vi "Untitled 6 (SubVI).vi"(0 "Path":path, 1 "Dust ID":sgl, 5 "Upper Timestamp":timestamp, 7 "Velocity Limits":cluster{dbl, dbl}, 8 "Lower Timestamp":timestamp, 9 "Minimun Session Quality":i8, 13 "Use Timestamp":bool, 16 "Use Dust ID":bool, 17 "Dust Material":string) -> (20 "Results Output":string, 21 "Results Error/Debug":string, 25 "Request":string)   [LabVIEW 2015]
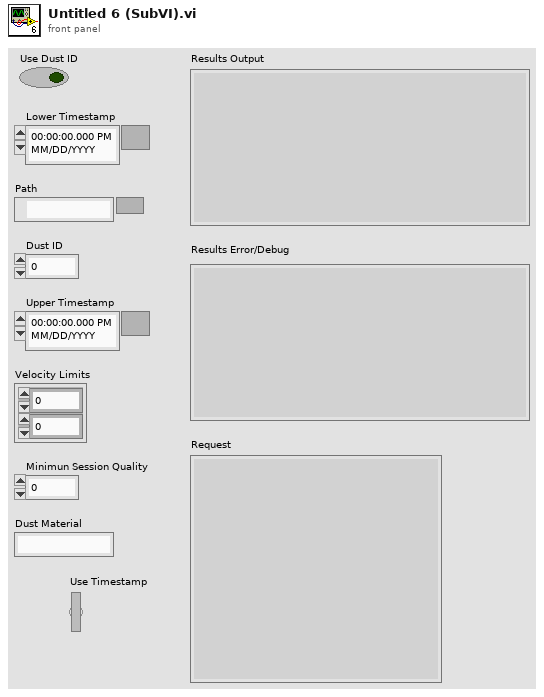
[diagram p1: front panel]
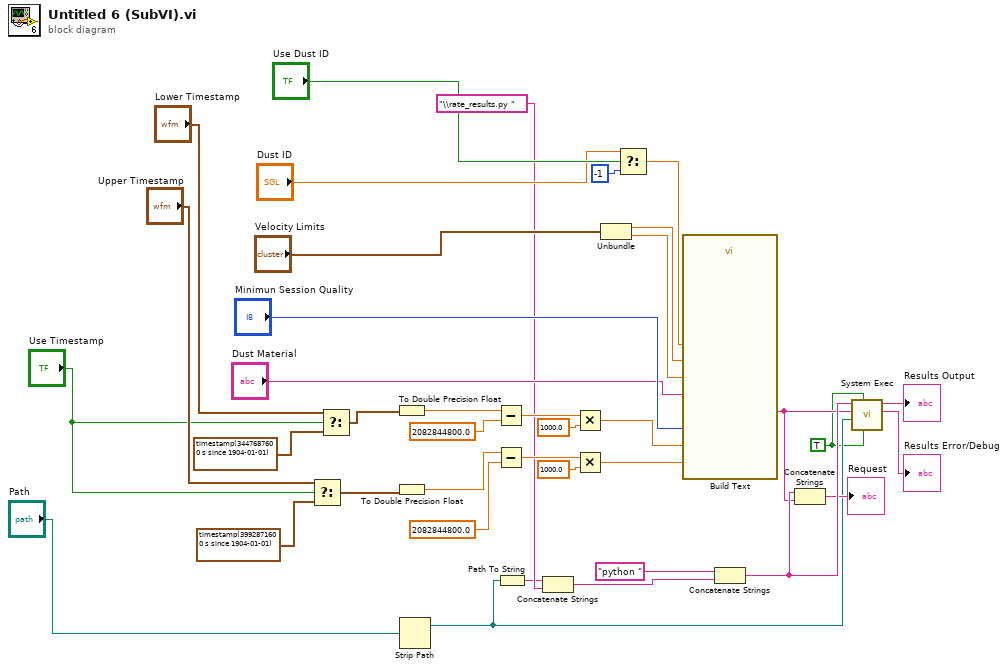
[diagram p0: block diagram]
diagram:
  w12 = TRUE
  n1 = Select(t="Upper Timestamp", s="Use Timestamp", f=timestamp(3992871600 s since 1904-01-01)) -> (s? t:f=w7:timestamp)
  n2 = Select(t="Lower Timestamp", s="Use Timestamp", f=timestamp(3447687600 s since 1904-01-01)) -> (s? t:f=w6:timestamp)
  n3 = To Double Precision Float(number=w6) -> (double precision float=w19:dbl)
  n4 = To Double Precision Float(number=w7) -> (double precision float=w15:dbl)
  n5 = Strip Path(path="Path") -> (stripped path=w13:path)  [unwired: 1 out]
  n6 = Subtract(x=w19, y=2082844800.0) -> (x-y=w21:dbl)
  n7 = Subtract(x=w15, y=2082844800.0) -> (x-y=w17:dbl)
  n8 = Path To String(path=w13) -> (string=w8:string)
  n9 = Concatenate Strings(w8, "\\rate_results.py ") -> (w11:string)
  n10 = Multiply(x=w21, y=1000.0) -> (x*y=w23:dbl)
  n11 = Multiply(x=w17, y=1000.0) -> (x*y=w24:dbl)
  n12 = Unbundle("Velocity Limits") -> (w26:dbl, w27:dbl)
  n13 = Select(t="Dust ID", s="Use Dust ID", f=-1) -> (s? t:f=w33:sgl)
  n14 = call "Build Text"("dustID"=w33, "vmax"=w27, "qual"="Minimun Session Quality", "start"=w23, "stop"=w24, "vmin"=w26, "material"="Dust Material") -> ("Result"=w35:string)  [unwired: 7 in, 1 out]
  n15 = Concatenate Strings("python ", w11) -> (w36:string)
  n16 = Concatenate Strings(w36, w35) -> (→"Request":string)
  n17 = call <vilib>:"System Exec.vi"("run minimized? (F)"=w12, "wait until completion? (T)"=w12, "working directory"=w13, "standard input"=w35, "command line"=w36) -> ("standard error"=→"Results Error/Debug":string, "standard output"=→"Results Output":string)  [unwired: 3 in, 2 out]
